vi "Convolucion_2.vi"() -> ()   [LabVIEW 2017]
panel:
  out "Tiempo 2":dbl[](array[numeric])
  out "Convolucion":dbl
  out "X2":dbl[](array[numeric])
  out "X1":dbl[](array[numeric])
  out "Tiempo":dbl[](array[numeric])
  in  "Vertical Fill Slide":dbl(slide) scale=-4.0..4.0
  out "XY Graph 3":cluster{"Tiempo":dbl[], "Areas":dbl[]}[](graph)
  out "XY Graph 2":cluster{dbl[], dbl[]}(graph)
  out "XY Graph":cluster{dbl[], dbl[]}(graph)
  in  "df":dbl
  in  "to":dbl
  in  "tf":dbl
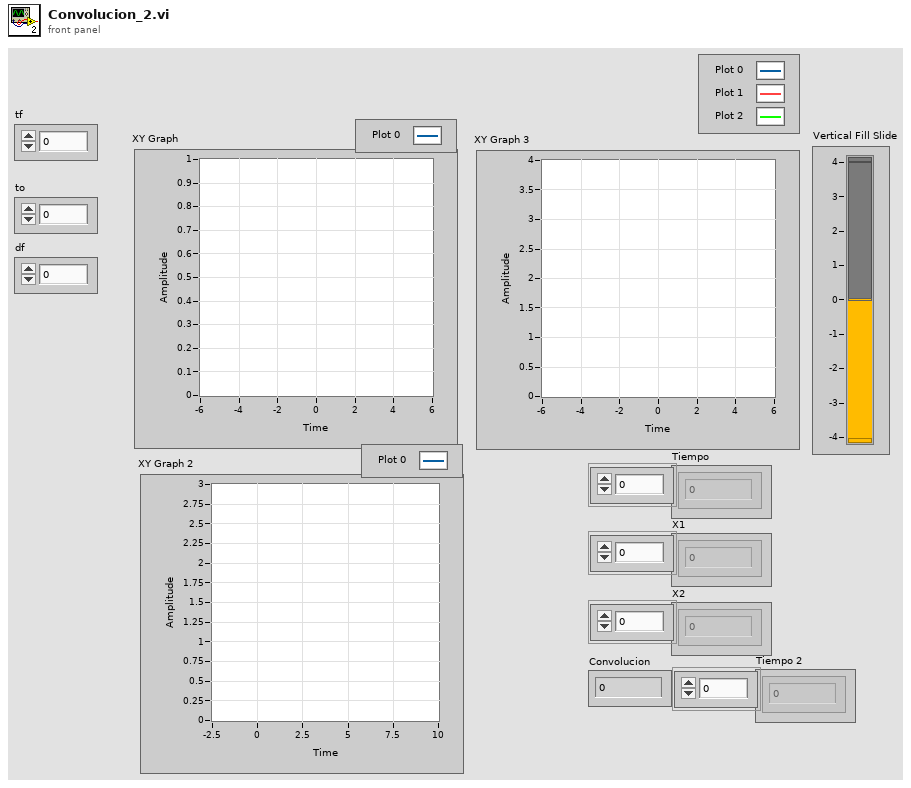
[diagram p1: front panel]
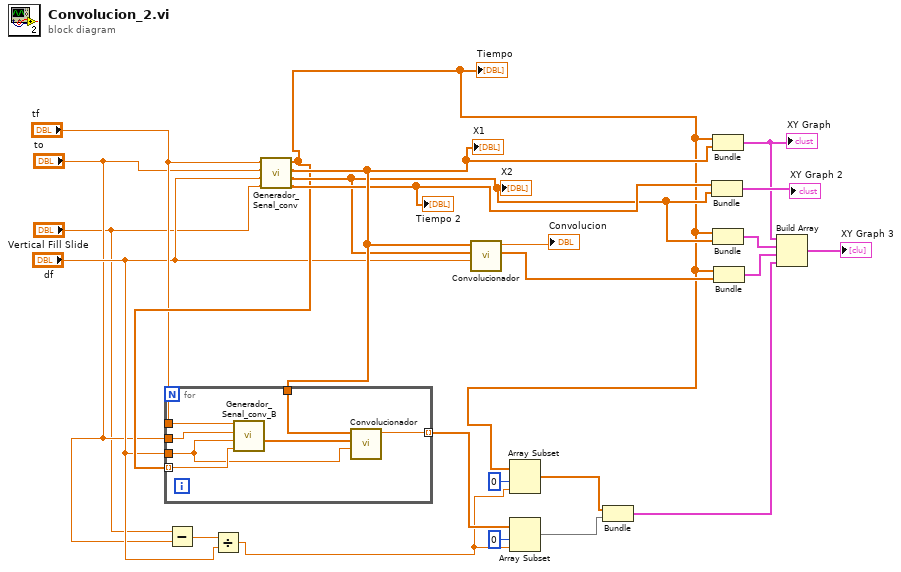
[diagram p0: block diagram]
diagram:
  n1 = Subtract(x="Vertical Fill Slide", y="to") -> (x-y=w9:dbl)
  n2 = Divide(x=w9, y="df") -> (x/y=w5:dbl)
  n3 = call "Generador_Senal_conv.vi"("Vertical Fill Slide"="Vertical Fill Slide", "df"="df", "to"="to", "tf"="tf") -> ("Tiempo 2"=w21:dbl[], "X2"=w19:dbl[], "X1"=w22:dbl[], "Tiempo"=w12:dbl[])  [unwired: 4 in]
  "Tiempo" <- w12
  "X1" <- w22
  "X2" <- w19
  "Tiempo 2" <- w21
  n4 = for {
    tunnel: w12 -> [w27] mode=indexing
    tunnel: "to" -> [w29]
    tunnel: "tf" -> [w28]
    tunnel: "df" -> [w26]
    tunnel: [w25] -> w11 mode=indexing
    tunnel: w22 -> [w24]
    n5 = call "Generador_Senal_conv_B.vi"("Vertical Fill Slide"=w27, "df"=w26, "to"=w29, "tf"=w28) -> ("X2"=w30:dbl[])  [unwired: 7 in]
    n6 = call "Convolucionador.vi"("df"=w26, "X2"=w30, "X1"=w24) -> ("Convolucion"=w25:dbl)  [unwired: 7 in, 1 out]
  }
  n7 = call "Convolucionador.vi"("df"="df", "X2"=w19, "X1"=w22) -> ("Areas"=w16:dbl[], "Convolucion"=→"Convolucion":dbl)  [unwired: 7 in]
  n8 = Array Subset(array=w12, index=0, length=w5) -> (w3:dbl[])
  n9 = Array Subset(array=w11, index=0, length=w5) -> (w2:dbl[])
  n10 = Bundle(w3, w2) -> (w13:cluster{dbl[], dbl[]})  [unwired: 1 in]
  n11 = Bundle("Tiempo 2"=w21, "X2"=w19) -> (→"XY Graph 2":cluster{"Tiempo 2":dbl[], "X2":dbl[]})  [unwired: 1 in]
  n12 = Bundle("Tiempo"=w12, "X1"=w22) -> (w18:cluster{"Tiempo":dbl[], "X1":dbl[]})  [unwired: 1 in]
  "XY Graph" <- w18
  n13 = Bundle("Tiempo"=w12, "X2"=w19) -> (w17:cluster{"Tiempo":dbl[], "X2":dbl[]})  [unwired: 1 in]
  n14 = Bundle("Tiempo"=w12, "Areas"=w16) -> (w15:cluster{"Tiempo":dbl[], "Areas":dbl[]})  [unwired: 1 in]
  n15 = Build Array(w18, w17, w15, w13) -> (→"XY Graph 3":cluster{"Tiempo":dbl[], "Areas":dbl[]}[])
